vi "Pre Launch Init.vi"(11 "Nested in":refnum<class "SIMULATED.lvclass">) -> (0 "error out":errorcluster, 3 "Nested out":refnum<class "SIMULATED.lvclass">)   [LabVIEW 2019, in "SIMULATED.lvclass"]
doc: "(<B>Filename</B>: Actor Framework.lvlib:Actor.lvclass:Pre Launch Init.vi)\n\nDefines behavior that occurs after the Launch Nested Actor method is invoked but before the actor's Actor Core method begins running.\n\nBy default, this method does nothing. A descendant class may override it to define behavior."
uses:
  SIMULATED.lvclass
  Serial Devices/Serial Devices.lvclass
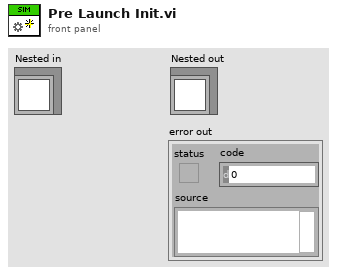
[diagram p1: front panel]
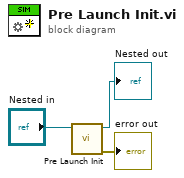
[diagram p0: block diagram]
diagram:
  n1 = call-parent "Pre Launch Init.vi"("Nested in"="Nested in") -> ("error out"=→"error out":errorcluster, "Nested out"=→"Nested out":refnum<class "SIMULATED.lvclass">)  [unwired: 9 in]
